vi "CalcLR.vi"(2 "Right":dbl[](array[numeric]), 3 "Left":dbl[](array[numeric])) -> (0 "Right":dbl, 1 "Left":dbl)   [LabVIEW 2016]
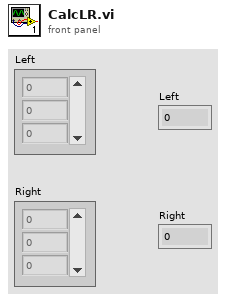
[diagram p1: front panel]
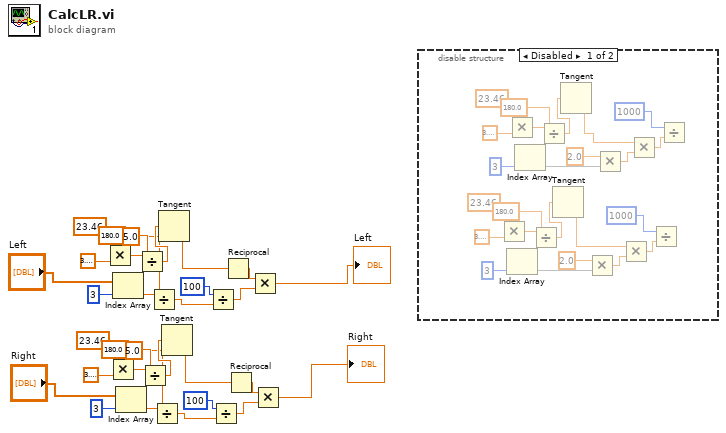
[diagram p0: block diagram]
diagram:
  n1 = Multiply(x=23.46, y=3.141592653589793) -> (x*y=w28:dbl)
  n2 = Multiply(x=23.46, y=3.141592653589793) -> (x*y=w13:dbl)
  n3 = Index Array(array="Left", index=3) -> (element=w22:dbl)
  n4 = Index Array(array="Right", index=3) -> (element=w8:dbl)
  n5 = Divide(x=w28, y=180.0) -> (x/y=w26:dbl)
  n6 = Divide(x=w13, y=180.0) -> (x/y=w11:dbl)
  n7 = Divide(x=w22, y=5.0) -> (x/y=w19:dbl)
  n8 = Divide(x=w8, y=5.0) -> (x/y=w1:dbl)
  n9 = Tangent(1:w26) -> (0:w23:dbl)
  n10 = Tangent(1:w11) -> (0:w9:dbl)
  n11 = Divide(x=100, y=w19) -> (x/y=w18:dbl)
  n12 = Divide(x=100, y=w1) -> (x/y=w5:dbl)
  n13 = Reciprocal(x=w23) -> (1/x=w17:dbl)
  n14 = Reciprocal(x=w9) -> (1/x=w4:dbl)
  n15 = Multiply(x=w17, y=w18) -> (x*y=→"Left":dbl)
  n16 = Multiply(x=w4, y=w5) -> (x*y=→"Right":dbl)
  n17 = disable-structure shown="Disabled" {
    frame Disabled {
      n18 = Multiply(x=23.46, y=3.141592653589793) -> (x*y=w44:dbl)
      n19 = Multiply(x=23.46, y=3.141592653589793) -> (x*y=w55:dbl)
      n20 = Index Array(index=3) -> (array=w33:dbl[], element=w40)
      n21 = Index Array(index=3) -> (array=w32:dbl[], element=w51)
      n22 = Divide(x=w44, y=180.0) -> (x/y=w42:dbl)
      n23 = Divide(x=w55, y=180.0) -> (x/y=w53:dbl)
      n24 = Tangent(1:w42) -> (0:w35:dbl)
      n25 = Tangent(1:w53) -> (0:w34:dbl)
      n26 = Multiply(x=2.0, y=w40) -> (x*y=w38:dbl)
      n27 = Multiply(x=2.0, y=w51) -> (x*y=w49:dbl)
      n28 = Multiply(x=w35, y=w38) -> (x*y=w37:dbl)
      n29 = Multiply(x=w34, y=w49) -> (x*y=w48:dbl)
      n30 = Divide(x=1000, y=w37) -> ()  [unwired: 1 out]
      n31 = Divide(x=1000, y=w48) -> (x/y=w31:dbl)
    }
    frame Enabled {
    }
  }
